vi "Found Target2.vi"() -> (3 "Boolean":bool)   [LabVIEW 2016]
uses:
  <vilib>/Rock Robotics/Network Tables/NT Read Number.vi
  <vilib>/Rock Robotics/Network Tables/NT Read Boolean.vi
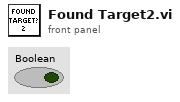
[diagram p1: front panel]
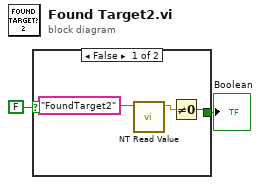
[diagram p0: block diagram]
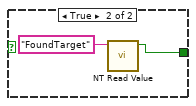
[diagram p2: hidden frame]
diagram:
  n1 = case shown="False" FALSE {
    tunnel: [w3 w7] -> w2
    frame False {
      n2 = call-poly <vilib>:"NT Read Value.vi"("Name"="FoundTarget2") -> ("Numeric"=w4:dbl)  [unwired: 9 in, 1 out]
      n3 = Not Equal To 0?(x=w4) -> (x != 0?=w3:bool)
    }
    frame True {
      n4 = call-poly <vilib>:"NT Read Value.vi"("Name"="FoundTarget") -> ("Boolean"=w7:bool)  [unwired: 9 in, 1 out]
    }
  }
  "Boolean" <- w2
